vi "Build DashBoard Data.vi"(11 "Dashboard Enables":T3={"Analog Module 1"=[TRUE, TRUE, TRUE, TRUE, TRUE, TRUE, TRUE, TRUE], "Analog Module 2"=[FALSE, FALSE, FALSE, FALSE, FALSE, FALSE, FALSE, FALSE], "Digital Module 1"=TRUE, "Digital Module 2"=FALSE, "Solenoid Module"=TRUE}) -> ()   [LabVIEW 2011]
doc: "This VI builds data and sends it back to the dashboard PC program. By default it sends back the raw values for the first analog, digital, and solenoid module. Modify it to send back the data you want to view. Consider adding higher level data to the Dashboard Datatype.ctl and to this VI. Then update the Dashboard to display the data however you like.\n\nThis software is licensed. Open the labview\\readme\\WPI Robotics Library Open Source License.txt file for more information."
uses:
  DashboardEnable.ctl
  Dashboard Datatype.ctl
  <vilib>/Rock Robotics/WPI/DriverStation/WPI_DriverStationDigitalData.ctl
  Robot Global Data.vi
panel:
  out "Dashboard Data":T1
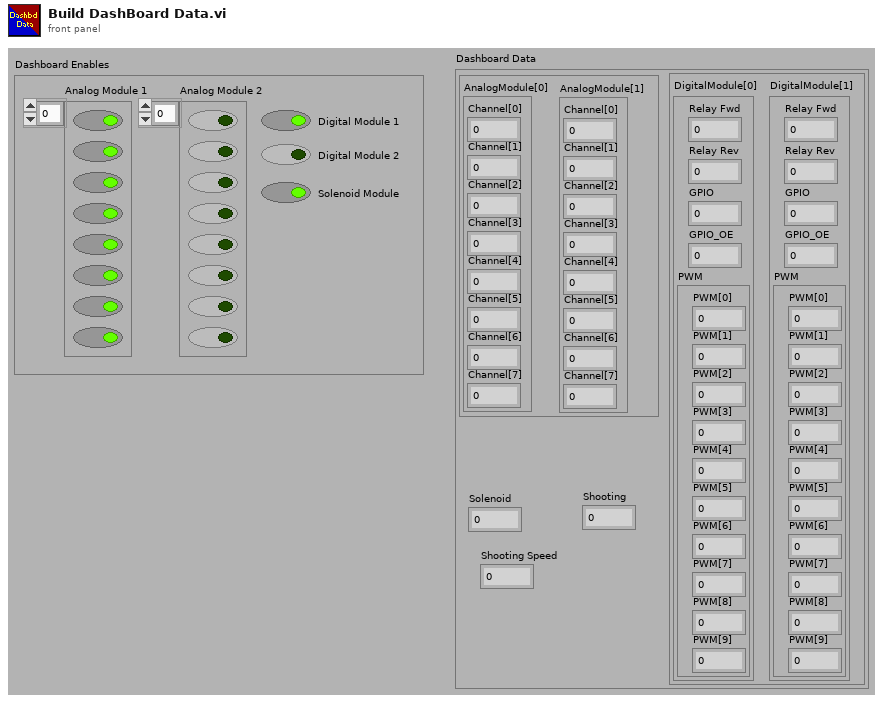
[diagram p1: front panel]
types:
  T1 = typedef "Dashboard Datatype.ctl" = cluster{cluster{"AnalogModule[0]":cluster{"Channel[0]":sgl, "Channel[1]":sgl, "Channel[2]":sgl, "Channel[3]":sgl, "Channel[4]":sgl, "Channel[5]":sgl, "Channel[6]":sgl, "Channel[7]":sgl}, "AnalogModule[1]":cluster{"Channel[0]":sgl, "Channel[1]":sgl, "Channel[2]":sgl, "Channel[3]":sgl, "Channel[4]":sgl, "Channel[5]":sgl, "Channel[6]":sgl, "Channel[7]":sgl}}, cluster{"DigitalModule[0]":T2, "DigitalModule[1]":T2}, "Solenoid":u8, "Shooting":dbl, "Shooting Speed":dbl}
  T2 = typedef "WPI_DriverStationDigitalData.ctl" = cluster{"Relay Fwd":u8, "Relay Rev":u8, "GPIO":u16, "GPIO_OE":u16, "PWM":cluster{"PWM[0]":u8, "PWM[1]":u8, "PWM[2]":u8, "PWM[3]":u8, "PWM[4]":u8, "PWM[5]":u8, "PWM[6]":u8, "PWM[7]":u8, "PWM[8]":u8, "PWM[9]":u8}}
  T3 = typedef "DashboardEnable.ctl" = cluster{"Analog Module 1":bool[], "Analog Module 2":bool[], "Digital Module 1":bool, "Digital Module 2":bool, "Solenoid Module":bool}
  T4 = cluster{"AnalogModule[0]":cluster{"Channel[0]":sgl, "Channel[1]":sgl, "Channel[2]":sgl, "Channel[3]":sgl, "Channel[4]":sgl, "Channel[5]":sgl, "Channel[6]":sgl, "Channel[7]":sgl}, "AnalogModule[1]":cluster{"Channel[0]":sgl, "Channel[1]":sgl, "Channel[2]":sgl, "Channel[3]":sgl, "Channel[4]":sgl, "Channel[5]":sgl, "Channel[6]":sgl, "Channel[7]":sgl}}
  T5 = cluster{"Channel[0]":sgl, "Channel[1]":sgl, "Channel[2]":sgl, "Channel[3]":sgl, "Channel[4]":sgl, "Channel[5]":sgl, "Channel[6]":sgl, "Channel[7]":sgl}[]
  T6 = cluster{"Channel[0]":sgl, "Channel[1]":sgl, "Channel[2]":sgl, "Channel[3]":sgl, "Channel[4]":sgl, "Channel[5]":sgl, "Channel[6]":sgl, "Channel[7]":sgl}
  T7 = cluster{"AnalogModule[0][0]":sgl, "AnalogModule[0][1]":sgl, "AnalogModule[0][2]":sgl, "AnalogModule[0][3]":sgl, "AnalogModule[0][4]":sgl, "AnalogModule[0][5]":sgl, "AnalogModule[0][6]":sgl, "AnalogModule[0][7]":sgl}
  T8 = cluster{"[0]":cluster{"Channel[0]":sgl, "Channel[1]":sgl, "Channel[2]":sgl, "Channel[3]":sgl, "Channel[4]":sgl, "Channel[5]":sgl, "Channel[6]":sgl, "Channel[7]":sgl}, "[1]":cluster{"Channel[0]":sgl, "Channel[1]":sgl, "Channel[2]":sgl, "Channel[3]":sgl, "Channel[4]":sgl, "Channel[5]":sgl, "Channel[6]":sgl, "Channel[7]":sgl}}
  T9 = cluster{"DigitalModule[0]":T2, "DigitalModule[1]":T2}
  T10 = typedef "FPGA_DIODevRef.ctl" = cluster{"DevStatus":errorcluster, "Module":T11}
  T11 = typedef "FPGA_TypedefDigitalModule.ctl" = enum16{"Digital Module 1", "Digital Module 2"}
  T12 = cluster{"[0]":u8, "[1]":u8, "[2]":u8, "[3]":u8, "[4]":u8, "[5]":u8, "[6]":u8, "[7]":u8, "[8]":u8, "[9]":u8}
  T13 = typedef "FPGA_SolenoidDevRef.ctl" = cluster{"DevStatus":errorcluster, "Module":T14}
  T14 = typedef "FPGA_TypedefSolenoidModule.ctl" = enum16{"Solenoid Module 1", "Solenoid Module 2"}
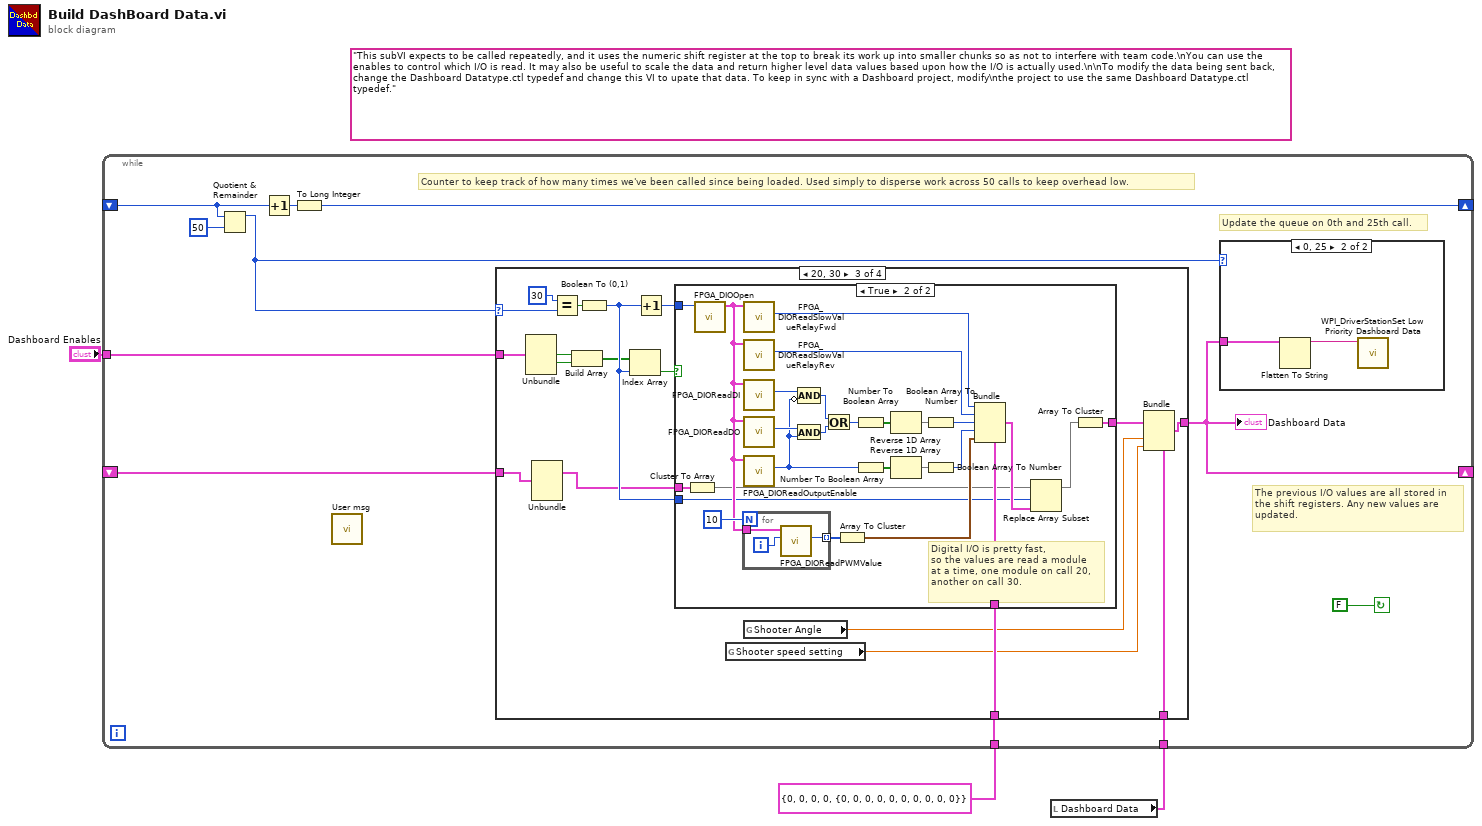
[diagram p0: block diagram]
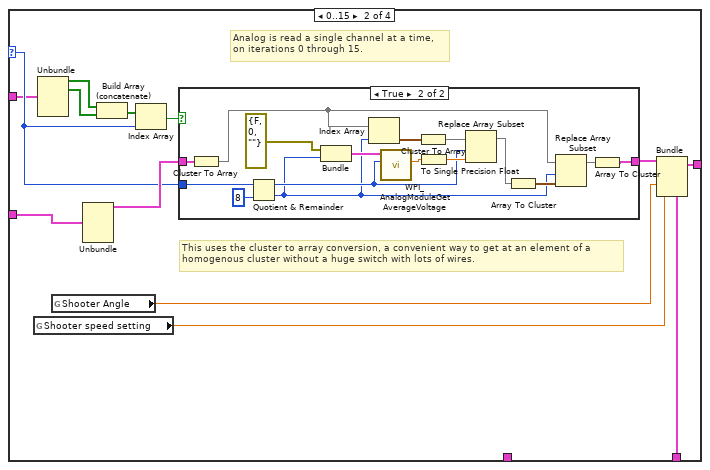
[diagram p4: hidden frame]
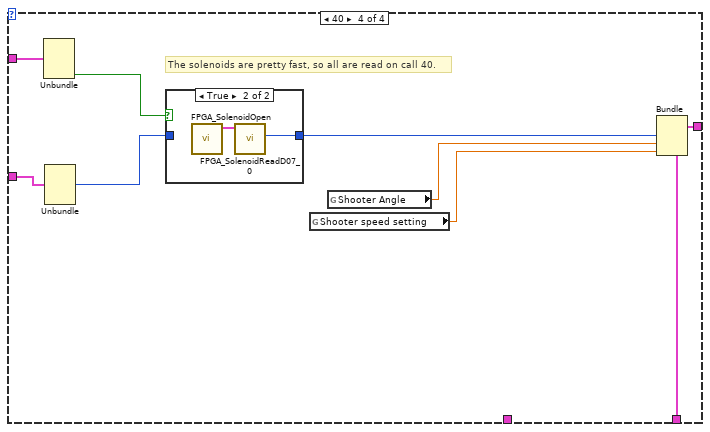
[diagram p7: hidden frame]
diagram:
  (unwired) "This subVI expects to be called repeatedly, and it uses the numeric shift register at the top to break its work up into smaller chunks so as not to interfere with team code.\nYou can use the enables to control which I/O is read. It may also be useful to scale the data and return higher level data values based upon how the I/O is actually used.\n\nTo modify the data being sent back, change the Dashboard Datatype.ctl typedef and change this VI to upate that data. To keep in sync with a Dashboard project, modify\nthe project to use the same Dashboard Datatype.ctl typedef."
  n1 = local read "Dashboard Data"() -> (w2:T1)
  n2 = while {
    shift-right: [w7] -> _
    shift-left: _ -> [w9]
    shift-right: [w4] -> _
    shift-left: _ -> [w12]
    tunnel: T2 {"Relay Fwd"=0, "Relay Rev"=0, "GPIO"=0, "GPIO_OE"=0, "PWM"={"PWM[0]"=0, "PWM[1]"=0, "PWM[2]"=0, "PWM[3]"=0, "PWM[4]"=0, "PWM[5]"=0, "PWM[6]"=0, "PWM[7]"=0, "PWM[8]"=0, "PWM[9]"=0}} ("DigitalModule[1]") -> [w11]
    tunnel: w2 -> [w6]
    tunnel: "Dashboard Enables" -> [w5]
    stop <- FALSE continue-if-true
    # "Counter to keep track of how many times we've been called since being loaded. Used simply to disperse work across 50 calls to keep overhead low."
    # "Update the queue on 0th and 25th call."
    # "The previous I/O values are all stored in\nthe shift registers. Any new values are\nupdated."
    n3 = Quotient & Remainder(x=w9, y=50) -> (x-y*floor(x/y)=w8:i32)  [unwired: 1 out]
    n4 = Increment(x=w9) -> (x+1=w14:i32)
    n5 = To Long Integer(number=w14) -> (32bit integer=w7:i32)
    n6 = call "User msg.vi"() -> ()  [unwired: 12 in]
    n7 = case shown="20, 30" w8 {
      selector: w8 -> [_ w25 w59 _]
      tunnel: [w17 w21 w50 w101] -> w4
      tunnel: w12 -> [w17 w20 w52 w103]
      tunnel: w11 -> [_ _ w65 _]
      tunnel: w6 -> [_ w27 w51 w100]
      tunnel: w5 -> [_ w24 w57 w104]
      frame Default {
        # "Don't update any I/O"
      }
      frame 0..15 {
        # "This uses the cluster to array conversion, a convenient way to get at an element of a\nhomogenous cluster without a huge switch with lots of wires."
        # "Analog is read a single channel at a time,\non iterations 0 through 15."
        n8 = global read "Robot Global Data.vi" "Shooter speed setting"() -> (w18:dbl)
        n9 = Unbundle(w24) -> ("Analog Module 1"=w23:bool[], "Analog Module 2"=w22:bool[])  [unwired: 3 out]
        n10 = global read "Robot Global Data.vi" "Shooter Angle"() -> (w19:dbl)
        n11 = Unbundle(w20) -> (w26:T4)  [unwired: 4 out]
        n12 = Build Array (concatenate)(w23, w22) -> (w29:bool[])
        n13 = Index Array(array=w29, index=w25) -> (element=w30:bool)
        n14 = case shown="True" w30 {
          tunnel: w25 -> [_ w38]
          tunnel: [w31 w35] -> w28
          tunnel: w26 -> [w31 w34]
          frame False {
          }
          frame True {
            n15 = Cluster To Array(cluster=w34) -> (array=w33:T5)
            n16 = Quotient & Remainder(x=w38, y=8) -> (x-y*floor(x/y)=w37:i32, floor(x/y)=w32:i32)
            n17 = Bundle("DevStatus"=errorcluster {"status"=FALSE, "code"=0, "source"=""}, w32) -> (w46:cluster{"DevStatus":errorcluster, i32})  [unwired: 1 out]
            n18 = Index Array(array=w33, index=w32) -> (element=w40:T6)
            n19 = call <vilib>:"WPI_AnalogModuleGetAverageVoltage.vi"("Channel"=w37, "AnalogModuleDevStatus"=w46) -> ("Average Voltage"=w43:dbl)  [unwired: 1 in, 8 out]
            n20 = Cluster To Array(cluster=w40) -> (array=w39:sgl[])
            n21 = To Single Precision Float(number=w43) -> (single precision float=w42:sgl)
            n22 = Replace Array Subset(array=w39, new element=w42, index=w37) -> (w41:sgl[])
            n23 = Array To Cluster(array=w41) -> (cluster=w45:T7)
            n24 = Replace Array Subset(array=w33, new element=w45, index=w32) -> (w36:T5)
            n25 = Array To Cluster(array=w36) -> (cluster=w35:T8)
          }
        }
        n26 = Bundle(cluster=w27, w28, "Shooting"=w19, "Shooting Speed"=w18) -> (w21:T1)  [unwired: 2 out]
      }
      frame 20, 30 {
        n27 = Unbundle(w57) -> ("Digital Module 1"=w56:bool, "Digital Module 2"=w55:bool)  [unwired: 3 out]
        n28 = Unbundle(w52) -> (w54:T9)  [unwired: 4 out]
        n29 = Equal?(x=30, y=w59) -> (x = y?=w63:bool)
        n30 = Build Array(w56, w55) -> (w58:bool[])
        n31 = Boolean To (0,1)(Boolean=w63) -> (0, 1=w61:i16)
        n32 = Index Array(array=w58, index=w61) -> (element=w60:bool)
        n33 = Increment(x=w61) -> (x+1=w62:i16)
        n34 = case shown="True" w60 {
          tunnel: w65 -> [_ w74]
          tunnel: [w66 w67] -> w53
          tunnel: w62 -> [_ w72]
          tunnel: w61 -> [_ w71]
          tunnel: w54 -> [w66 w70]
          frame False {
          }
          frame True {
            # "Digital I/O is pretty fast,\nso the values are read a module\nat a time, one module on call 20,\nanother on call 30."
            n35 = Cluster To Array(cluster=w70) -> (array=w69:T2[])
            n36 = call <vilib>:"FPGA_DIOOpen.vi"("Module (Module 1)"=w72) -> ("DIODeviceRef"=w90:T10)  [unwired: 1 in, 9 out]
            n37 = for {
              N: 10 -> [_]
              tunnel: w90 -> [w95]
              tunnel: [w93] -> w91 mode=indexing
              i -> [w94]
              n38 = call <vilib>:"FPGA_DIOReadPWMValue.vi"("PWMChannel"=w94, "DIODeviceRef In"=w95) -> ("PWMValue"=w93:u8)  [unwired: 1 in, 8 out]
            }
            n39 = call <vilib>:"FPGA_DIOReadSlowValueRelayFwd.vi"("DIODeviceRef In"=w90) -> ("Relay Forward"=w83:u8)  [unwired: 1 in, 9 out]
            n40 = call <vilib>:"FPGA_DIOReadSlowValueRelayRev.vi"("DIODeviceRef In"=w90) -> ("Relay Reverse"=w84:u8)  [unwired: 1 in, 9 out]
            n41 = call <vilib>:"FPGA_DIOReadDI.vi"("DIODeviceRef In"=w90) -> ("DI"=w88:u16)  [unwired: 1 in, 9 out]
            n42 = call <vilib>:"FPGA_DIOReadDO.vi"("DIODeviceRef In"=w90) -> ("DO"=w87:u16)  [unwired: 1 in, 9 out]
            n43 = call <vilib>:"FPGA_DIOReadOutputEnable.vi"("DIODeviceRef In"=w90) -> ("OutputEnable"=w78:u16)  [unwired: 1 in, 9 out]
            n44 = And(x=w87, y=w78) -> (x .and. y?=w86:u16)
            n45 = Compound Arithmetic op=AND(w88, invert w78) -> (w85:u16)
            n46 = Or(x=w85, y=w86) -> (x .or. y?=w76:u16)
            n47 = Array To Cluster(array=w91) -> (cluster=w89:T12)
            n48 = Number To Boolean Array(number=w76) -> (Boolean array=w81:bool[])
            n49 = Number To Boolean Array(number=w78) -> (Boolean array=w80:bool[])
            n50 = Reverse 1D Array(array=w81) -> (reversed array=w82:bool[])
            n51 = Reverse 1D Array(array=w80) -> (reversed array=w79:bool[])
            n52 = Boolean Array To Number(Boolean array=w82) -> (number=w75:u32)
            n53 = Boolean Array To Number(Boolean array=w79) -> (number=w77:u32)
            n54 = Bundle(cluster=w74, "Relay Fwd"=w83, "Relay Rev"=w84, "GPIO"=w75, "GPIO_OE"=w77, "PWM"=w89) -> (w73:T2)
            n55 = Replace Array Subset(array=w69, new element=w73, index=w71) -> (w68:T2[])
            n56 = Array To Cluster(array=w68) -> (cluster=w67:cluster{"[0]":T2, "[1]":T2})
          }
        }
        n57 = global read "Robot Global Data.vi" "Shooter speed setting"() -> (w48:dbl)
        n58 = global read "Robot Global Data.vi" "Shooter Angle"() -> (w49:dbl)
        n59 = Bundle(cluster=w51, w53, "Shooting"=w49, "Shooting Speed"=w48) -> (w50:T1)  [unwired: 2 out]
      }
      frame 40 {
        # "The solenoids are pretty fast, so all are read on call 40."
        n60 = Unbundle(w104) -> ("Solenoid Module"=w98:bool)  [unwired: 4 out]
        n61 = Unbundle(w103) -> ("Solenoid"=w102:u8)  [unwired: 4 out]
        n62 = case shown="True" w98 {
          tunnel: [w105 w106] -> w99
          tunnel: w102 -> [w105 _]
          frame False {
          }
          frame True {
            n63 = call <vilib>:"FPGA_SolenoidOpen.vi"() -> ("SolenoidDevRef"=w107:T13)  [unwired: 2 in, 9 out]
            n64 = call <vilib>:"FPGA_SolenoidReadD07_0.vi"("SolenoidDevRef"=w107) -> ("DO7:0"=w106:u8)  [unwired: 1 in, 9 out]
          }
        }
        n65 = global read "Robot Global Data.vi" "Shooter speed setting"() -> (w96:dbl)
        n66 = global read "Robot Global Data.vi" "Shooter Angle"() -> (w97:dbl)
        n67 = Bundle(cluster=w100, "Solenoid"=w99, "Shooting"=w97, "Shooting Speed"=w96) -> (w101:T1)  [unwired: 2 out]
      }
    }
    "Dashboard Data" <- w4
    n68 = case shown="0, 25" w8 {
      tunnel: w4 -> [_ w16]
      frame Default {
      }
      frame 0, 25 {
        n69 = Flatten To String(anything=w16) -> (data string=w15:string)  [unwired: 1 in, 4 out]
        n70 = call <vilib>:"WPI_DriverStationSet Low Priority Dashboard Data.vi"("User Data"=w15) -> ()  [unwired: 1 in, 10 out]
      }
    }
  }
